vi "IBM4_Diff_Read(IN).vi"(7 "Number":i32=10 min=1, 8 "error in":errorcluster, 9 "Neg-Chan":enum16{"A2", "A3", "A4", "A5"}(ring)=enum."A3", 10 "Pos-Chan":enum16{"A2", "A3", "A4", "A5"}(ring), 11 "COM resource in":refnum<visa-resource-name>="COM9") -> (0 "error out":errorcluster, 2 "array":i32[](array[numeric]), 3 "COM resource out":refnum<visa-resource-name>)   [LabVIEW 2023, in "IBM4.lvlib"]
doc: "This VI interfaces with the IBM4 to perform a differential read operation.\n\nThe number of readings should be greater than zero. At some point the number of reading will be too high and will cause a timeout error. This should only happen for numbers larger than 10000. The output will be an array of integer values.\n\nAlternate read operations exist covering binary or floating point, single reading, multiple readings, and an average of multiple readings (floating point only)."
uses:
  <instrlib>/IBM4/IBM4.lvlib
  <vilib>/regexp/Match Regular Expression.xnode
panel:
  out "error out 2":errorcluster
  out "read buffer":string
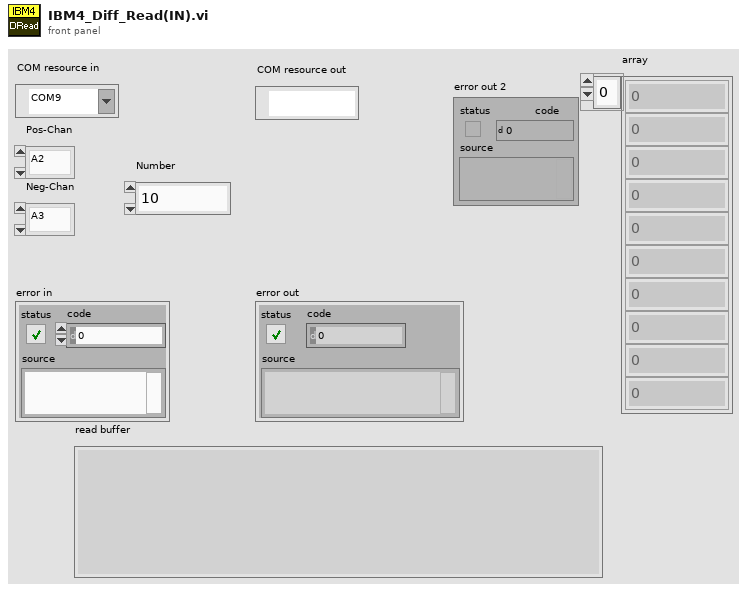
[diagram p1: front panel]
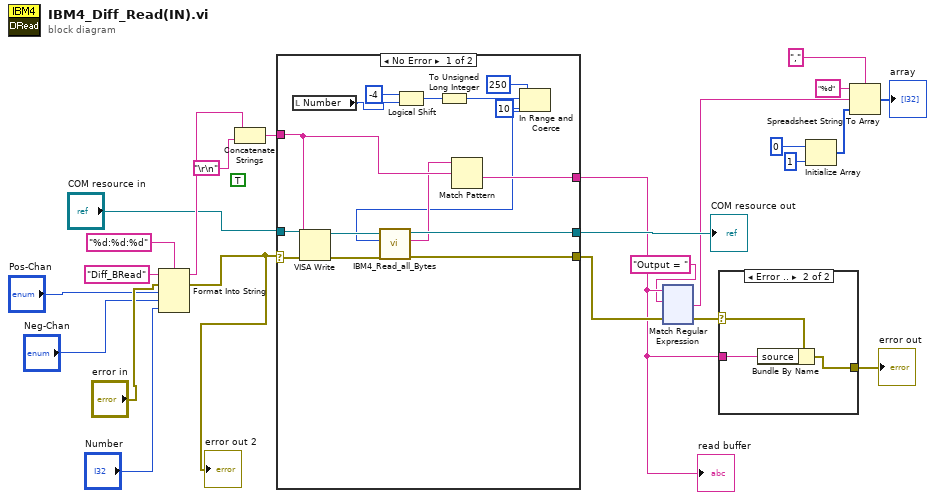
[diagram p0: block diagram]
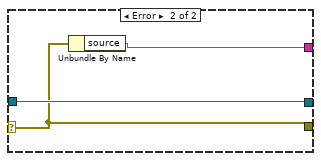
[diagram p3: hidden frame]
diagram:
  (unwired) TRUE ("Enable Termination\nChar (T)")
  n1 = Format Into String(format string="%d:%d:%d", initial string="Diff_BRead", error in="error in", "Pos-Chan", "Neg-Chan", "Number") -> (resulting string=w19:string, error out=w3:errorcluster)
  "error out 2" <- w3
  n2 = Concatenate Strings(w19, "\r\n") -> (w18:string)
  n3 = case shown="No Error" w3 {
    selector: w3 -> [w37 w41]
    tunnel: "COM resource in" -> [w40 w43]
    tunnel: [w35 w41] -> w9
    tunnel: [w39 w42] -> w7
    tunnel: w18 -> [w38 _]
    tunnel: [w36 w43] -> w21
    frame No Error {
      n4 = local read "Number"() -> (w28:i32)
      n5 = VISA Write(VISA resource name=w40, write buffer=w38, error in (no error)=w37) -> (VISA resource name out=w27:refnum<visa-resource-name>, error out=w26:errorcluster)  [unwired: 1 out]
      n6 = Logical Shift(y=i16 -4, x=w28) -> (x << y=w31:i32)
      n7 = To Unsigned Long Integer(number=w31) -> (unsigned 32bit integer=w29:u32)
      n8 = In Range and Coerce(upper limit=u32 250, x=w29, lower limit=u32 10) -> (coerced(x)=w25:u32)  [unwired: 1 out]
      n9 = call <instrlib>:"IBM4_Read_all_Bytes.vi"("error in (no error)"=w26, "milliseconds to wait"=w25, "VISA Refnum in"=w27) -> ("error out"=w35:errorcluster, "String"=w34:string, "VISA Refnum out"=w36:refnum<visa-resource-name>)  [unwired: 2 in]
      n10 = Match Pattern(string=w34, regular expression=w38) -> (after substring=w39:string)  [unwired: 1 in, 3 out]
    }
    frame Error {
      n11 = Unbundle By Name(w41) -> ("source"=w42:string)
    }
  }
  "COM resource out" <- w21
  "read buffer" <- w7
  n12 = xnode "Match Regular Expression"("input string"=w7, "regular expression"="Output = " ("format string"), "error in"=w9) -> ("after match"=w5:string, "error out"=w8:errorcluster)  [unwired: 3 in, 3 out]
  n13 = case shown="Error .." w8 {
    selector: w8 -> [w44 w47]
    tunnel: [w44 w45] -> w17
    tunnel: w7 -> [_ w46]
    frame No Error {
    }
    frame Error {
      n14 = Bundle By Name(cluster=w47, "source"=w46) -> (w45:errorcluster)
    }
  }
  "error out" <- w17
  n15 = Initialize Array(0, 1 ("dimension size")) -> (w14:i32[])
  n16 = Spreadsheet String To Array(delimiter (Tab)=",", format string="%d", spreadsheet string=w5, array type (2D Dbl)=w14) -> (array=→"array":i32[])
